vi "Copy Host to SCM Data.vi"(5 "Files Generated by Build":path[](array[path]), 6 "Top Level/Always Included VIs":path[](array[path]), 7 "Destination Path":path, 8 "error in (no error)":errorcluster, 9 "Target Name":string, 10 "Build Specification Name":string, 11 "Project Path":path) -> (0 "error out":errorcluster)   [LabVIEW 2015]
doc: "This VI is called after each run of a build specification. The VI will copy the generated LLB (Engine or System Explorer) into the VeriStand Custom Device folder (...\\Documents\\National Instruments\\NI VeriStand 2013...)."
uses:
  <vilib>/Utility/sysdir.llb/System Directory Type.ctl
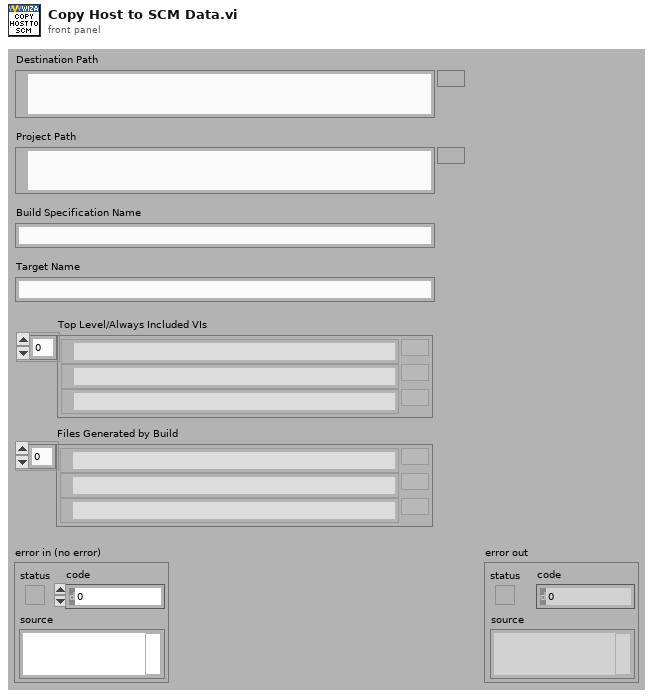
[diagram p1: front panel]
types:
  T1 = typedef "System Directory Type.ctl" = i32
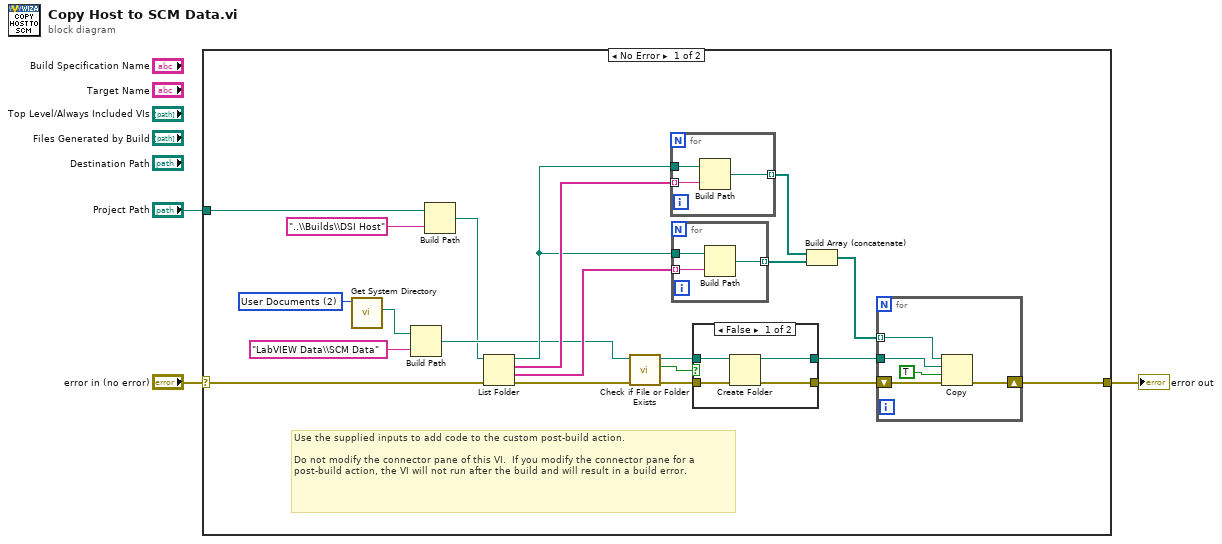
[diagram p0: block diagram]
diagram:
  n1 = case shown="No Error" "error in (no error)" {
    selector: "error in (no error)" -> [w5 w42]
    tunnel: [w12 w42] -> w2
    tunnel: "Project Path" -> [w8 _]
    frame No Error {
      w13 = T1 2 items=["User Home"=0, "User Desktop"=1, "User Documents"=2, "User Application Data"=3, "User Preferences"=4, "User Temporary"=5, "Public Documents"=6, "Public Application Data"=7, "Public Preferences"=8, "Public Cache"=13, "System Core Libraries"=9, "System Installed Libraries"=10, "Application Files"=11, "Boot Volume Root"=12] ("system directory type")
      # "Use the supplied inputs to add code to the custom post-build action.\n\nDo not modify the connector pane of this VI.  If you modify the connector pane for a post-build action, the VI will not run after the build and will result in a build error."
      n2 = call <vilib>:"Get System Directory.vi"("system directory type"=w13) -> ("system directory"=w14:path)  [unwired: 10 in]
      n3 = Build Path(base path=w14, name or relative path="LabVIEW Data\\SCM Data") -> (appended path=w11:path)
      n4 = Build Path(base path=w8, name or relative path="..\\Builds\\DSI Host") -> (appended path=w4:path)
      n5 = List Folder(path=w4, error in=w5) -> (path out=w17:path, filenames=w24:string[], folder names=w18:string[], error out=w15:errorcluster)  [unwired: 2 in]
      n6 = call <vilib>:"Check if File or Folder Exists.vi"("error in (no error)"=w15, "path"=w11) -> ("error out"=w19:errorcluster, "file or folder exists?"=w21:bool, "dup path"=w20:path)  [unwired: 7 in]
      n7 = for {
        tunnel: w24 -> [w40] mode=indexing
        tunnel: w17 -> [w41]
        tunnel: [w39] -> w23 mode=indexing
        n8 = Build Path(base path=w41, name or relative path=w40) -> (appended path=w39:path)
      }
      n9 = for {
        tunnel: w18 -> [w37] mode=indexing
        tunnel: w17 -> [w38]
        tunnel: [w36] -> w16 mode=indexing
        n10 = Build Path(base path=w38, name or relative path=w37) -> (appended path=w36:path)
      }
      n11 = case shown="False" w21 {
        tunnel: w20 -> [w28 w30]
        tunnel: w19 -> [w27 w29]
        tunnel: [w26 w30] -> w10
        tunnel: [w25 w29] -> w9
        frame False {
          n12 = Create Folder(path (use dialog)=w28, error in=w27) -> (created path=w26:path, error out=w25:errorcluster)  [unwired: 1 in, 1 out]
        }
        frame True {
        }
      }
      n13 = Build Array (concatenate)(w23, w16) -> (w22:path[])
      n14 = for {
        tunnel: w22 -> [w32] mode=indexing
        shift-right: [w33] -> w12
        shift-left: w9 -> [w34]
        tunnel: w10 -> [w31]
        n15 = Copy(8:w34, 9:TRUE ("overwrite (F)"), 10:w31, 11:w32) -> (0:w33:errorcluster)  [unwired: 1 in, 2 out]
      }
    }
    frame Error {
    }
  }
  "error out" <- w2
